vi "rsscope_core_global.vi"() -> ()   [LabVIEW 2014] (continued)
"Descriptive Name"="Search ARINC429 Label Data SSM", "Data Type"=0, "Command"="SEAR:TRIG:ARIN:SSM", "Access"=1, "Range Table"="", "Read Callback"="", "Write Callback"="rsscope_FormatSearchNameInt32_WriteCallback.vi", "Supported Models"="RTO|RTP", "Instrument Options"="", "Flags"=0, "Help"="Sets the sign/status matrix (SSM) bits.\n\nAvailable Repeated Capabilities:\nNone\n\nRemote-control command(s):\nSEARch:TRIGger:ARINc:SSM"}, {"Level"=5, "Class Only"=FALSE, "Identifier"="RSSCOPE_ATTR_SEARCH_ARINC429_LABEL_PATTERN_CONDITION", "Descriptive Name"="Search ARINC429 Label Pattern Condition", "Data Type"=0, "Command"="SEAR:TRIG:ARIN:LAB:COND", "Access"=2, "Range Table"="rsscope_rngProtocolARINC429LabelOperator", "Read Callback"="rsscope_FormatSearchNameInt32_ReadCallback.vi", "Write Callback"="rsscope_FormatSearchNameInt32_WriteCallback.vi", "Supported Models"="RTO|RTP", "Instrument Options"="", "Flags"=0, "Help"="Sets the condition for the label. You can define an exact label or a label range.\n\nAvailable Repeated Capabilities:\nNone\n\nRemote-control command(s):\nSEARch:TRIGger:ARINc:LABel:CONDition"}, {"Level"=5, "Class Only"=FALSE, "Identifier"="RSSCOPE_ATTR_SEARCH_ARINC429_LABEL_PATTERN_MIN", "Descriptive Name"="Search ARINC429 Label Pattern Min", "Data Type"=2, "Command"="SEAR:TRIG:ARIN:LAB:MIN", "Access"=1, "Range Table"="", "Read Callback"="", "Write Callback"="rsscope_FormatSearchNameString_WriteCallback.vi", "Supported Models"="RTO|RTP", "Instrument Options"="", "Flags"=0, "Help"="Defines the minimum bit pattern for the label.\n\nAvailable Repeated Capabilities:\nNone\n\nRemote-control command(s):\nSEARch:TRIGger:ARINc:LABel:MIN"}, {"Level"=5, "Class Only"=FALSE, "Identifier"="RSSCOPE_ATTR_SEARCH_ARINC429_LABEL_PATTERN_MAX", "Descriptive Name"="Search ARINC429 Label Pattern Max", "Data Type"=2, "Command"="SEAR:TRIG:ARIN:LAB:MAX", "Access"=1, "Range Table"="", "Read Callback"="", "Write Callback"="rsscope_FormatSearchNameString_WriteCallback.vi", "Supported Models"="RTO|RTP", "Instrument Options"="", "Flags"=0, "Help"="Sets the end value of a label pattern if &apos;Label Pattern Condition&apos; is set to InRange or OutOfRange.\n\nAvailable Repeated Capabilities:\nNone\n\nRemote-control command(s):\nSEARch:TRIGger:ARINc:LABel:MAX"}, {"Level"=5, "Class Only"=FALSE, "Identifier"="RSSCOPE_ATTR_SEARCH_ARINC429_DATA_PATTERN_CONDITION", "Descriptive Name"="Search ARINC429 Data Pattern Condition", "Data Type"=0, "Command"="SEAR:TRIG:ARIN:DATA:COND", "Access"=2, "Range Table"="rsscope_rngProtocolARINC429DataOperator", "Read Callback"="rsscope_FormatSearchNameInt32_ReadCallback.vi", "Write Callback"="rsscope_FormatSearchNameInt32_WriteCallback.vi", "Supported Models"="RTO|RTP", "Instrument Options"="", "Flags"=0, "Help"="Sets the condition for the data. You can define an exact data patterm or a data range.\n\nAvailable Repeated Capabilities:\nNone\n\nRemote-control command(s):\nSEARch:TRIGger:ARINc:DATA:CONDition"}, {"Level"=5, "Class Only"=FALSE, "Identifier"="RSSCOPE_ATTR_SEARCH_ARINC429_DATA_PATTERN_MIN", "Descriptive Name"="Search ARINC429 Data Pattern Min", "Data Type"=2, "Command"="SEAR:TRIG:ARIN:DATA:MIN", "Access"=1, "Range Table"="", "Read Callback"="", "Write Callback"="rsscope_FormatSearchNameString_WriteCallback.vi", "Supported Models"="RTO|RTP", "Instrument Options"="", "Flags"=0, "Help"="Defines the minimum bit pattern for the data.\n\nAvailable Repeated Capabilities:\nNone\n\nRemote-control command(s):\nSEARch:TRIGger:ARINc:DATA:MIN"}, {"Level"=5, "Class Only"=FALSE, "Identifier"="RSSCOPE_ATTR_SEARCH_ARINC429_DATA_PATTERN_MAX", "Descriptive Name"="Search ARINC429 Data Pattern Max", "Data Type"=2, "Command"="SEAR:TRIG:ARIN:DATA:MAX", "Access"=1, "Range Table"="", "Read Callback"="", "Write Callback"="rsscope_FormatSearchNameString_WriteCallback.vi", "Supported Models"="RTO|RTP", "Instrument Options"="", "Flags"=0, "Help"="Sets the end value of a data pattern if &apos;Data Pattern Condition&apos; is set to InRange or OutOfRange.\n\nAvailable Repeated Capabilities:\nNone\n\nRemote-control command(s):\nSEARch:TRIGger:ARINc:DATA:MAX"}, {"Level"=4, "Class Only"=TRUE, "Identifier"="", "Descriptive Name"="Error Condition", "Data Type"=0, "Command"="", "Access"=0, "Range Table"="", "Read Callback"="", "Write Callback"="", "Supported Models"="", "Instrument Options"="", "Flags"=0, "Help"="Specifies the error conditions to be searched for."}, {"Level"=5, "Class Only"=FALSE, "Identifier"="RSSCOPE_ATTR_SEARCH_ARINC429_ERROR_CODING_ERROR", "Descriptive Name"="Search ARINC429 Error Coding Error", "Data Type"=3, "Command"="SEAR:TRIG:ARIN:ERR:COD", "Access"=2, "Range Table"="", "Read Callback"="rsscope_FormatSearchNameBoolean_ReadCallback.vi", "Write Callback"="rsscope_FormatSearchNameBoolean_WriteCallback.vi", "Supported Models"="RTO|RTP", "Instrument Options"="", "Flags"=0, "Help"="Enables search when a coding error occurs.\n\nAvailable Repeated Capabilities:\nNone\n\nRemote-control command(s):\nSEARch:TRIGger:ARINc:ERRor:CODing"}, {"Level"=5, "Class Only"=FALSE, "Identifier"="RSSCOPE_ATTR_SEARCH_ARINC429_ERROR_PARITY_ERROR", "Descriptive Name"="Search ARINC429 Error Parity Error", "Data Type"=3, "Command"="SEAR:TRIG:ARIN:ERR:PAR", "Access"=2, "Range Table"="", "Read Callback"="rsscope_FormatSearchNameBoolean_ReadCallback.vi", "Write Callback"="rsscope_FormatSearchNameBoolean_WriteCallback.vi", "Supported Models"="RTO|RTP", "Instrument Options"="", "Flags"=0, "Help"="Enables search when a parity error occurs.\n\nAvailable Repeated Capabilities:\nNone\n\nRemote-control command(s):\nSEARch:TRIGger:ARINc:ERRor:PARity"}, {"Level"=5, "Class Only"=FALSE, "Identifier"="RSSCOPE_ATTR_SEARCH_ARINC429_ERROR_TIMING_ERROR", "Descriptive Name"="Search ARINC429 Error Timing Error", "Data Type"=3, "Command"="SEAR:TRIG:ARIN:ERR:TIM", "Access"=2, "Range Table"="", "Read Callback"="rsscope_FormatSearchNameBoolean_ReadCallback.vi", "Write Callback"="rsscope_FormatSearchNameBoolean_WriteCallback.vi", "Supported Models"="RTO|RTP", "Instrument Options"="", "Flags"=0, "Help"="Enables the search for timing errors, when the minimum gap is out of range.\n\nAvailable Repeated Capabilities:\nNone\n\nRemote-control command(s):\nSEARch:TRIGger:ARINc:ERRor:TIMing"}, {"Level"=4, "Class Only"=TRUE, "Identifier"="", "Descriptive Name"="Results", "Data Type"=0, "Command"="", "Access"=0, "Range Table"="", "Read Callback"="", "Write Callback"="", "Supported Models"="", "Instrument Options"="", "Flags"=0, "Help"="Returns the search of the specified word."}, {"Level"=5, "Class Only"=FALSE, "Identifier"="RSSCOPE_ATTR_SEARCH_ARINC429_WORDS_COUNT", "Descriptive Name"="Search ARINC429 Words Count", "Data Type"=0, "Command"="SEAR:RES:ARIN:WCO?", "Access"=0, "Range Table"="", "Read Callback"="rsscope_FormatSearchNameInt32_ReadCallback.vi", "Write Callback"="", "Supported Models"="RTO|RTP", "Instrument Options"="", "Flags"=0, "Help"="Returns the number of decoded words.\n\nAvailable Repeated Capabilities:\nNone\n\nRemote-control command(s):\nSEARch:RESult:ARINc:WCOunt?"}, {"Level"=3, "Class Only"=TRUE, "Identifier"="", "Descriptive Name"="RFFE", "Data Type"=0, "Command"="", "Access"=0, "Range Table"="", "Read Callback"="", "Write Callback"="", "Supported Models"="", "Instrument Options"="", "Flags"=0, "Help"="Configures RFFE search settings."}, {"Level"=4, "Class Only"=FALSE, "Identifier"="RSSCOPE_ATTR_SEARCH_RFFE_TYPE", "Descriptive Name"="Search RFFE Type", "Data Type"=0, "Command"="SEAR:TRIG:RFFE:TYPE", "Access"=2, "Range Table"="rsscope_rngProtocolRFFETriggerType", "Read Callback"="rsscope_FormatSearchNameInt32_ReadCallback.vi", "Write Callback"="rsscope_FormatSearchNameInt32_WriteCallback.vi", "Supported Models"="", "Instrument Options"="K40", "Flags"=0, "Help"="Sets the event to be searched for.\n\nAvailable Repeated Capabilities:\nNone\n\nRemote-control command(s):\nSEARch:TRIGger:RFFE:TYPE"}, {"Level"=4, "Class Only"=FALSE, "Identifier"="RSSCOPE_ATTR_SEARCH_RFFE_INTERRUPT_PATTERN", "Descriptive Name"="Search RFFE Interrupt Pattern", "Data Type"=2, "Command"="SEAR:TRIG:RFFE:INT", "Access"=2, "Range Table"="", "Read Callback"="rsscope_FormatSearchNameString_ReadCallback.vi", "Write Callback"="rsscope_FormatSearchNameString_WriteCallback.vi", "Supported Models"="", "Instrument Options"="K40", "Flags"=0, "Help"="Defines the pattern of the interrrupt identification sequence, which consists of interrupt slots 15 to 0.\n\nAvailable Repeated Capabilities:\nNone\n\nRemote-control command(s):\nSEARch:TRIGger:RFFE:INTerrupt"}, {"Level"=4, "Class Only"=TRUE, "Identifier"="", "Descriptive Name"="Slave Address", "Data Type"=0, "Command"="", "Access"=0, "Range Table"="", "Read Callback"="", "Write Callback"="", "Supported Models"="", "Instrument Options"="", "Flags"=0, "Help"="Searches for a slave address or a slave address range."}, {"Level"=5, "Class Only"=FALSE, "Identifier"="RSSCOPE_ATTR_SEARCH_RFFE_SLAVE_CONDITION", "Descriptive Name"="Search RFFE Slave Condition", "Data Type"=0, "Command"="SEAR:TRIG:RFFE:SADD:COND", "Access"=2, "Range Table"="rsscope_rngProtocolTriggerCondition", "Read Callback"="rsscope_FormatSearchNameInt32_ReadCallback.vi", "Write Callback"="rsscope_FormatSearchNameInt32_WriteCallback.vi", "Supported Models"="", "Instrument Options"="K40", "Flags"=0, "Help"="Sets the operator to search for a specific pattern or a range\n\nAvailable Repeated Capabilities:\nNone\n\nRemote-control command(s):\nSEARch:TRIGger:RFFE:SADD:CONDition"}, {"Level"=5, "Class Only"=FALSE, "Identifier"="RSSCOPE_ATTR_SEARCH_RFFE_SLAVE_MIN", "Descriptive Name"="Search RFFE Slave Min", "Data Type"=2, "Command"="SEAR:TRIG:RFFE:SADD:MIN", "Access"=1, "Range Table"="", "Read Callback"="", "Write Callback"="rsscope_FormatSearchNameString_WriteCallback.vi", "Supported Models"="", "Instrument Options"="K40", "Flags"=0, "Help"="Specifies a pattern, or sets the start value of a pattern range.\n\nAvailable Repeated Capabilities:\nNone\n\nRemote-control command(s):\nSEARch:TRIGger:RFFE:SADD:MIN"}, {"Level"=5, "Class Only"=FALSE, "Identifier"="RSSCOPE_ATTR_SEARCH_RFFE_SLAVE_MAX", "Descriptive Name"="Search RFFE Slave Max", "Data Type"=2, "Command"="SEAR:TRIG:RFFE:SADD:MAX", "Access"=1, "Range Table"="", "Read Callback"="", "Write Callback"="rsscope_FormatSearchNameString_WriteCallback.vi", "Supported Models"="", "Instrument Options"="K40", "Flags"=0, "Help"="Sets the end value of an range if the corresponding condition is set to In Range or Out Of Range.\n\nAvailable Repeated Capabilities:\nNone\n\nRemote-control command(s):\nSEARch:TRIGger:RFFE:SADD:MAX"}, {"Level"=4, "Class Only"=TRUE, "Identifier"="", "Descriptive Name"="Address", "Data Type"=0, "Command"="", "Access"=0, "Range Table"="", "Read Callback"="", "Write Callback"="", "Supported Models"="", "Instrument Options"="", "Flags"=0, "Help"="Searches for a register address or an address range."}, {"Level"=5, "Class Only"=FALSE, "Identifier"="RSSCOPE_ATTR_SEARCH_RFFE_ADDRESS_CONDITION", "Descriptive Name"="Search RFFE Address Condition", "Data Type"=0, "Command"="SEAR:TRIG:RFFE:ADDR:COND", "Access"=2, "Range Table"="rsscope_rngProtocolTriggerCondition", "Read Callback"="rsscope_FormatSearchNameInt32_ReadCallback.vi", "Write Callback"="rsscope_FormatSearchNameInt32_WriteCallback.vi", "Supported Models"="", "Instrument Options"="K40", "Flags"=0, "Help"="Sets the operator to search for a specific pattern or a range\n\nAvailable Repeated Capabilities:\nNone\n\nRemote-control command(s):\nSEARch:TRIGger:RFFE:ADDRess:CONDition"}, {"Level"=5, "Class Only"=FALSE, "Identifier"="RSSCOPE_ATTR_SEARCH_RFFE_ADDRESS_MIN", "Descriptive Name"="Search RFFE Address Min", "Data Type"=2, "Command"="SEAR:TRIG:RFFE:ADDR:MIN", "Access"=1, "Range Table"="", "Read Callback"="", "Write Callback"="rsscope_FormatSearchNameString_WriteCallback.vi", "Supported Models"="", "Instrument Options"="K40", "Flags"=0, "Help"="Specifies a pattern, or sets the start value of a pattern range.\n\nAvailable Repeated Capabilities:\nNone\n\nRemote-control command(s):\nSEARch:TRIGger:RFFE:ADDRess:MIN"}, {"Level"=5, "Class Only"=FALSE, "Identifier"="RSSCOPE_ATTR_SEARCH_RFFE_ADDRESS_MAX", "Descriptive Name"="Search RFFE Address Max", "Data Type"=2, "Command"="SEAR:TRIG:RFFE:ADDR:MAX", "Access"=1, "Range Table"="", "Read Callback"="", "Write Callback"="rsscope_FormatSearchNameString_WriteCallback.vi", "Supported Models"="", "Instrument Options"="K40", "Flags"=0, "Help"="Sets the end value of an range if the corresponding condition is set to In Range or Out Of Range.\n\nAvailable Repeated Capabilities:\nNone\n\nRemote-control command(s):\nSEARch:TRIGger:RFFE:ADDRess:MAX"}, {"Level"=4, "Class Only"=TRUE, "Identifier"="", "Descriptive Name"="Byte Count", "Data Type"=0, "Command"="", "Access"=0, "Range Table"="", "Read Callback"="", "Write Callback"="", "Supported Models"="", "Instrument Options"="", "Flags"=0, "Help"="Searches for a byte count or a byte count range."}, {"Level"=5, "Class Only"=FALSE, "Identifier"="RSSCOPE_ATTR_SEARCH_RFFE_BYTE_COUNT_CONDITION", "Descriptive Name"="Search RFFE Byte Count Condition", "Data Type"=0, "Command"="SEAR:TRIG:RFFE:BCO:COND", "Access"=2, "Range Table"="rsscope_rngProtocolTriggerCondition", "Read Callback"="rsscope_FormatSearchNameInt32_ReadCallback.vi", "Write Callback"="rsscope_FormatSearchNameInt32_WriteCallback.vi", "Supported Models"="", "Instrument Options"="K40", "Flags"=0, "Help"="Sets the operator to search for a specific pattern or a range\n\nAvailable Repeated Capabilities:\nNone\n\nRemote-control command(s):\nSEARch:TRIGger:RFFE:BCOunt:CONDition"}, {"Level"=5, "Class Only"=FALSE, "Identifier"="RSSCOPE_ATTR_SEARCH_RFFE_BYTE_COUNT_MIN", "Descriptive Name"="Search RFFE Byte Count Min", "Data Type"=2, "Command"="SEAR:TRIG:RFFE:BCO:MIN", "Access"=1, "Range Table"="", "Read Callback"="", "Write Callback"="rsscope_FormatSearchNameString_WriteCallback.vi", "Supported Models"="", "Instrument Options"="K40", "Flags"=0, "Help"="Specifies a pattern, or sets the start value of a pattern range.\n\nAvailable Repeated Capabilities:\nNone\n\nRemote-control command(s):\nSEARch:TRIGger:RFFE:BCOunt:MIN"}, {"Level"=5, "Class Only"=FALSE, "Identifier"="RSSCOPE_ATTR_SEARCH_RFFE_BYTE_COUNT_MAX", "Descriptive Name"="Search RFFE Byte Count Max", "Data Type"=2, "Command"="SEAR:TRIG:RFFE:BCO:MAX", "Access"=1, "Range Table"="", "Read Callback"="", "Write Callback"="rsscope_FormatSearchNameString_WriteCallback.vi", "Supported Models"="", "Instrument Options"="K40", "Flags"=0, "Help"="Sets the end value of an range if the corresponding condition is set to In Range or Out Of Range.\n\nAvailable Repeated Capabilities:\nNone\n\nRemote-control command(s):\nSEARch:TRIGger:RFFE:BCOunt:MAX"}, {"Level"=4, "Class Only"=TRUE, "Identifier"="", "Descriptive Name"="Data", "Data Type"=0, "Command"="", "Access"=0, "Range Table"="", "Read Callback"="", "Write Callback"="", "Supported Models"="", "Instrument Options"="", "Flags"=0, "Help"="Searches for a data pattern or an data word range."}, {"Level"=5, "Class Only"=FALSE, "Identifier"="RSSCOPE_ATTR_SEARCH_RFFE_DATA_CONDITION", "Descriptive Name"="Search RFFE Data Condition", "Data Type"=0, "Command"="SEAR:TRIG:RFFE:DATA:DCON", "Access"=2, "Range Table"="rsscope_rngProtocolTriggerCondition", "Read Callback"="rsscope_FormatSearchNameInt32_ReadCallback.vi", "Write Callback"="rsscope_FormatSearchNameInt32_WriteCallback.vi", "Supported Models"="", "Instrument Options"="K40", "Flags"=0, "Help"="Sets the operator to search for a specific pattern or a range\n\nAvailable Repeated Capabilities:\nNone\n\nRemote-control command(s):\nSEARch:TRIGger:RFFE:DATA:DCON"}, {"Level"=5, "Class Only"=FALSE, "Identifier"="RSSCOPE_ATTR_SEARCH_RFFE_DATA_MIN", "Descriptive Name"="Search RFFE Data Min", "Data Type"=2, "Command"="SEAR:TRIG:RFFE:DATA:DMIN", "Access"=1, "Range Table"="", "Read Callback"="", "Write Callback"="rsscope_FormatSearchNameString_WriteCallback.vi", "Supported Models"="", "Instrument Options"="K40", "Flags"=0, "Help"="Specifies a pattern, or sets the start value of a pattern range.\n\nAvailable Repeated Capabilities:\nNone\n\nRemote-control command(s):\nSEARch:TRIGger:RFFE:DATA:DMIN"}, {"Level"=5, "Class Only"=FALSE, "Identifier"="RSSCOPE_ATTR_SEARCH_RFFE_DATA_MAX", "Descriptive Name"="Search RFFE Data Max", "Data Type"=2, "Command"="SEAR:TRIG:RFFE:DATA:DMAX", "Access"=1, "Range Table"="", "Read Callback"="", "Write Callback"="rsscope_FormatSearchNameString_WriteCallback.vi", "Supported Models"="", "Instrument Options"="K40", "Flags"=0, "Help"="Sets the end value of an range if the corresponding condition is set to In Range or Out Of Range.\n\nAvailable Repeated Capabilities:\nNone\n\nRemote-control command(s):\nSEARch:TRIGger:RFFE:DATA:DMAX"}, {"Level"=4, "Class Only"=TRUE, "Identifier"="", "Descriptive Name"="Index", "Data Type"=0, "Command"="", "Access"=0, "Range Table"="", "Read Callback"="", "Write Callback"="", "Supported Models"="", "Instrument Options"="", "Flags"=0, "Help"="Defines which data frames are relevant for the search. The setting is available for all &apos;Extended Register&apos; command sequences, which can transfer more than one data frame. To search for any data byte that fulfills the data pattern settings, set the index to XX."}, {"Level"=5, "Class Only"=FALSE, "Identifier"="RSSCOPE_ATTR_SEARCH_RFFE_INDEX_CONDITION", "Descriptive Name"="Search RFFE Index Condition", "Data Type"=0, "Command"="SEAR:TRIG:RFFE:DATA:ICON", "Access"=2, "Range Table"="rsscope_rngProtocolIndexCondition", "Read Callback"="rsscope_FormatSearchNameInt32_ReadCallback.vi", "Write Callback"="rsscope_FormatSearchNameInt32_WriteCallback.vi", "Supported Models"="", "Instrument Options"="K40", "Flags"=0, "Help"="Sets the operator to search for a specific pattern or a range\n\nAvailable Repeated Capabilities:\nNone\n\nRemote-control command(s):\nSEARch:TRIGger:RFFE:DATA:ICON"}, {"Level"=5, "Class Only"=FALSE, "Identifier"="RSSCOPE_ATTR_SEARCH_RFFE_INDEX_MIN", "Descriptive Name"="Search RFFE Index Min", "Data Type"=0, "Command"="SEAR:TRIG:RFFE:DATA:IMIN", "Access"=2, "Range Table"="", "Read Callback"="rsscope_FormatSearchNameInt32_ReadCallback.vi", "Write Callback"="rsscope_FormatSearchNameInt32_WriteCallback.vi", "Supported Models"="", "Instrument Options"="K40", "Flags"=0, "Help"="Specifies a pattern, or sets the start value of a pattern range.\n\nAvailable Repeated Capabilities:\nNone\n\nRemote-control command(s):\nSEARch:TRIGger:RFFE:DATA:IMIN"}, {"Level"=5, "Class Only"=FALSE, "Identifier"="RSSCOPE_ATTR_SEARCH_RFFE_INDEX_MAX", "Descriptive Name"="Search RFFE Index Max", "Data Type"=0, "Command"="SEAR:TRIG:RFFE:DATA:IMAX", "Access"=2, "Range Table"="", "Read Callback"="rsscope_FormatSearchNameInt32_ReadCallback.vi", "Write Callback"="rsscope_FormatSearchNameInt32_WriteCallback.vi", "Supported Models"="", "Instrument Options"="K40", "Flags"=0, "Help"="Sets the end value of an range if the corresponding condition is set to In Range or Out Of Range.\n\nAvailable Repeated Capabilities:\nNone\n\nRemote-control command(s):\nSEARch:TRIGger:RFFE:DATA:IMAX"}, {"Level"=4, "Class Only"=TRUE, "Identifier"="", "Descriptive Name"="Error Conditions", "Data Type"=0, "Command"="", "Access"=0, "Range Table"="", "Read Callback"="", "Write Callback"="", "Supported Models"="", "Instrument Options"="", "Flags"=0, "Help"="This class configures conditions for Error search."}, {"Level"=5, "Class Only"=FALSE, "Identifier"="RSSCOPE_ATTR_SEARCH_RFFE_ERROR_SCC", "Descriptive Name"="Search RFFE Error SCC", "Data Type"=3, "Command"="SEAR:TRIG:RFFE:ERR:SSC", "Access"=2, "Range Table"="", "Read Callback"="rsscope_FormatSearchNameBoolean_ReadCallback.vi", "Write Callback"="rsscope_FormatSearchNameBoolean_WriteCallback.vi", "Supported Models"="", "Instrument Options"="", "Flags"=0, "Help"="Enables the trigger on an SSC error - when no valid SSC sequence has been found after the idle time.\n\nAvailable Repeated Capabilities:\nNone\n\nRemote-control command(s):\nSEARch:TRIGger:RFFE:ERRor:SSC"}, {"Level"=5, "Class Only"=FALSE, "Identifier"="RSSCOPE_ATTR_SEARCH_RFFE_ERROR_LENGTH", "Descriptive Name"="Search RFFE Error Length", "Data Type"=3, "Command"="SEAR:TRIG:RFFE:ERR:LENG", "Access"=2, "Range Table"="", "Read Callback"="rsscope_FormatSearchNameBoolean_ReadCallback.vi", "Write Callback"="rsscope_FormatSearchNameBoolean_WriteCallback.vi", "Supported Models"="", "Instrument Options"="", "Flags"=0, "Help"="Enables the trigger on a length error - when an incorrect length of the command sequence has been found.\n\nAvailable Repeated Capabilities:\nNone\n\nRemote-control command(s):\nSEARch:TRIGger:RFFE:ERRor:LENGth"}, {"Level"=5, "Class Only"=FALSE, "Identifier"="RSSCOPE_ATTR_SEARCH_RFFE_ERROR_PARITY", "Descriptive Name"="Search RFFE Error Parity", "Data Type"=3, "Command"="SEAR:TRIG:RFFE:ERR:PAR", "Access"=2, "Range Table"="", "Read Callback"="rsscope_FormatSearchNameBoolean_ReadCallback.vi", "Write Callback"="rsscope_FormatSearchNameBoolean_WriteCallback.vi", "Supported Models"="", "Instrument Options"="", "Flags"=0, "Help"="Enables the trigger on incorrect parity bits.\n\nAvailable Repeated Capabilities:\nNone\n\nRemote-control command(s):\nSEARch:TRIGger:RFFE:ERRor:PARity"}, {"Level"=5, "Class Only"=FALSE, "Identifier"="RSSCOPE_ATTR_SEARCH_RFFE_ERROR_GAP_TIME", "Descriptive Name"="Search RFFE Error Gap Time", "Data Type"=3, "Command"="SEAR:TRIG:RFFE:ERR:GAP", "Access"=2, "Range Table"="", "Read Callback"="rsscope_FormatSearchNameBoolean_ReadCallback.vi", "Write Callback"="rsscope_FormatSearchNameBoolean_WriteCallback.vi", "Supported Models"="", "Instrument Options"="", "Flags"=0, "Help"="Enables the search for RFFE gap time error.\n\nAvailable Repeated Capabilities:\nNone\n\nRemote-control command(s):\nSEARch:TRIGger:RFFE:ERRor:GAP"}, {"Level"=5, "Class Only"=FALSE, "Identifier"="RSSCOPE_ATTR_SEARCH_RFFE_ERROR_VERSION", "Descriptive Name"="Search RFFE Error Version", "Data Type"=3, "Command"="SEAR:TRIG:RFFE:ERR:VERS", "Access"=2, "Range Table"="", "Read Callback"="rsscope_FormatSearchNameBoolean_ReadCallback.vi", "Write Callback"="rsscope_FormatSearchNameBoolean_WriteCallback.vi", "Supported Models"="", "Instrument Options"="", "Flags"=0, "Help"="Enables the search for RFFE vresion error.\n\nAvailable Repeated Capabilities:\nNone\n\nRemote-control command(s):\nSEARch:TRIGger:RFFE:ERRor:VERSion"}, {"Level"=4, "Class Only"=TRUE, "Identifier"="", "Descriptive Name"="Results", "Data Type"=0, "Command"="", "Access"=0, "Range Table"="", "Read Callback"="", "Write Callback"="", "Supported Models"="", "Instrument Options"="", "Flags"=0, "Help"="Returns the search result of the specified sequence."}, {"Level"=5, "Class Only"=FALSE, "Identifier"="RSSCOPE_ATTR_SEARCH_RFFE_SEQUENCE_COUNT", "Descriptive Name"="Search RFFE Sequence Count", "Data Type"=0, "Command"="SEAR:RES:RFFE:FCO?", "Access"=0, "Range Table"="", "Read Callback"="rsscope_FormatSearchNameInt32_ReadCallback.vi", "Write Callback"="", "Supported Models"="RTO|RTP", "Instrument Options"="", "Flags"=0, "Help"="Returns the number of command sequences in the current acquisition.\n\nAvailable Repeated Capabilities:\nNone\n\nRemote-control command(s):\nSEARch:RESult:RFFE:FCOunt?"}, {"Level"=3, "Class Only"=TRUE, "Identifier"="", "Descriptive Name"="MDIO", "Data Type"=0, "Command"="", "Access"=0, "Range Table"="", "Read Callback"="", "Write Callback"="", "Supported Models"="", "Instrument Options"="", "Flags"=0, "Help"="Configures MDIO search, option K55."}, {"Level"=4, "Class Only"=FALSE, "Identifier"="RSSCOPE_ATTR_SEARCH_MDIO_TYPE", "Descriptive Name"="Search MDIO Type", "Data Type"=0, "Command"="SEAR:TRIG:MDIO:TYPE", "Access"=2, "Range Table"="rsscope_rngProtocolMDIOTriggerType", "Read Callback"="rsscope_FormatSearchNameInt32_ReadCallback.vi", "Write Callback"="rsscope_FormatSearchNameInt32_WriteCallback.vi", "Supported Models"="", "Instrument Options"="K55", "Flags"=0, "Help"="Selects the search type for MDIO analysis.\n\nAvailable Repeated Capabilities:\nNone\n\nRemote-control command(s):\nSEARch:TRIGger:MDIO:TYPE"}, {"Level"=4, "Class Only"=FALSE, "Identifier"="RSSCOPE_ATTR_SEARCH_MDIO_START_CODE", "Descriptive Name"="Search MDIO Start Code", "Data Type"=0, "Command"="SEAR:TRIG:MDIO:ST", "Access"=2, "Range Table"="rsscope_rngProtocolMDIOTriggerStartCode", "Read Callback"="rsscope_FormatSearchNameInt32_ReadCallback.vi", "Write Callback"="rsscope_FormatSearchNameInt32_WriteCallback.vi", "Supported Models"="", "Instrument Options"="K55", "Flags"=0, "Help"="Selects the start of frame code of the frame pattern.\n\nAvailable Repeated Capabilities:\nNone\n\nRemote-control command(s):\nSEARch:TRIGger:MDIO:ST"}, {"Level"=4, "Class Only"=FALSE, "Identifier"="RSSCOPE_ATTR_SEARCH_MDIO_OPERATION_CODE", "Descriptive Name"="Search MDIO Operation Code", "Data Type"=0, "Command"="SEAR:TRIG:MDIO:FRAM", "Access"=2, "Range Table"="rsscope_rngProtocolMDIOTriggerOperationCode", "Read Callback"="rsscope_FormatSearchNameInt32_ReadCallback.vi", "Write Callback"="rsscope_FormatSearchNameInt32_WriteCallback.vi", "Supported Models"="", "Instrument Options"="K55", "Flags"=0, "Help"="Selects the Type of Frame code (or OP code, OpCode, operation code).\n\nAvailable Repeated Capabilities:\nNone\n\nRemote-control command(s):\nSEARch:TRIGger:MDIO:FRAMetype"}, {"Level"=4, "Class Only"=FALSE, "Identifier"="RSSCOPE_ATTR_SEARCH_MDIO_PHYSICAL_PORT_ADDRESS", "Descriptive Name"="Search MDIO Physical Port Address", "Data Type"=2, "Command"="SEAR:TRIG:MDIO:PHYS", "Access"=1, "Range Table"="", "Read Callback"="", "Write Callback"="rsscope_FormatSearchNameString_WriteCallback.vi", "Supported Models"="", "Instrument Options"="K55", "Flags"=0, "Help"="Sets the physical address (in Clause 22) or port address (in Clause 45) of the frame pattern (5 bits).\n\nAvailable Repeated Capabilities:\nNone\n\nRemote-control command(s):\nSEARch:TRIGger:MDIO:PHYS"}, {"Level"=4, "Class Only"=FALSE, "Identifier"="RSSCOPE_ATTR_SEARCH_MDIO_REGISTER_DEVICE_ADDRESS", "Descriptive Name"="Search MDIO Register Device Address", "Data Type"=2, "Command"="SEAR:TRIG:MDIO:REGI", "Access"=1, "Range Table"="", "Read Callback"="", "Write Callback"="rsscope_FormatSearchNameString_WriteCallback.vi", "Supported Models"="", "Instrument Options"="K55", "Flags"=0, "Help"="Sets the register address (in Clause 22) or device address (in Clause 45) of the frame pattern (5 bits); available only in search type &apos;Data&apos;.\n\nAvailable Repeated Capabilities:\nNone\n\nRemote-control command(s):\nSEARch:TRIGger:MDIO:REGI"}, {"Level"=4, "Class Only"=FALSE, "Identifier"="RSSCOPE_ATTR_SEARCH_MDIO_DATA_ADDRESS_PATTERN", "Descriptive Name"="Search MDIO Data Address Pattern", "Data Type"=2, "Command"="SEAR:TRIG:MDIO:DATA", "Access"=1, "Range Table"="", "Read Callback"="", "Write Callback"="rsscope_FormatSearchNameString_WriteCallback.vi", "Supported Models"="", "Instrument Options"="K55", "Flags"=0, "Help"="Defines the 16-bit payload data pattern (both in Clause 22 or Clause 45) or the address pattern (in Clause 45, only) to search for.\n\nAvailable Repeated Capabilities:\nNone\n\nRemote-control command(s):\nSEARch:TRIGger:MDIO:DATA"}, {"Level"=4, "Class Only"=TRUE, "Identifier"="", "Descriptive Name"="Results", "Data Type"=0, "Command"="", "Access"=0, "Range Table"="", "Read Callback"="", "Write Callback"="", "Supported Models"="", "Instrument Options"="", "Flags"=0, "Help"="Returns the search result of the specified word."}, {"Level"=5, "Class Only"=FALSE, "Identifier"="RSSCOPE_ATTR_SEARCH_MDIO_WORD_COUNT", "Descriptive Name"="Search MDIO Word Count", "Data Type"=0, "Command"="SEAR:RES:MDIO:WCO?", "Access"=0, "Range Table"="", "Read Callback"="rsscope_FormatSearchNameInt32_ReadCallback.vi", "Write Callback"="", "Supported Models"="", "Instrument Options"="K55", "Flags"=0, "Help"="Returns the number of decoded words.\n\nAvailable Repeated Capabilities:\nNone\n\nRemote-control command(s):\nSEARch:RESult:MDIO:WCOunt?"}, {"Level"=3, "Class Only"=TRUE, "Identifier"="", "Descriptive Name"="Ethernet", "Data Type"=0, "Command"="", "Access"=0, "Range Table"="", "Read Callback"="", "Write Callback"="", "Supported Models"="", "Instrument Options"="", "Flags"=0, "Help"="This class contains attributes that configure the  Ethernet protocol variants 10BASE-T and 100BASE-TX.\n\nAttributes in this class require option R&S RTO-K8."}, {"Level"=4, "Class Only"=FALSE, "Identifier"="RSSCOPE_ATTR_SEARCH_ETHERNET_FRAME_ENABLED", "Descriptive Name"="Search Ethernet Frame Enabled", "Data Type"=3, "Command"="SEAR:TRIG:ETH:FRAM:SEL", "Access"=2, "Range Table"="", "Read Callback"="rsscope_FormatSearchNameBoolean_ReadCallback.vi", "Write Callback"="rsscope_FormatSearchNameBoolean_WriteCallback.vi", "Supported Models"="", "Instrument Options"="K8", "Flags"=0, "Help"="Defines, whether a search within a frame shall be activated or not.\n\nAvailable Repeated Capabilities:\nNone\n\nRemote-control command(s):\nSEARch:TRIGger:ETHernet:FRAMe:SELect"}, {"Level"=4, "Class Only"=FALSE, "Identifier"="RSSCOPE_ATTR_SEARCH_ETHERNET_ERROR_ENABLED", "Descriptive Name"="Search Ethernet Error Enabled", "Data Type"=3, "Command"="SEAR:TRIG:ETH:ERR:SEL", "Access"=2, "Range Table"="", "Read Callback"="rsscope_FormatSearchNameBoolean_ReadCallback.vi", "Write Callback"="rsscope_FormatSearchNameBoolean_WriteCallback.vi", "Supported Models"="", "Instrument Options"="K8", "Flags"=0, "Help"="Defines, whether a search for an error condition shall be activated or not.\n\nAvailable Repeated Capabilities:\nNone\n\nRemote-control command(s):\nSEARch:TRIGger:ETHernet:ERRor:SELect"}, {"Level"=4, "Class Only"=TRUE, "Identifier"="", "Descriptive Name"="Destination Address", "Data Type"=0, "Command"="", "Access"=0, "Range Table"="", "Read Callback"="", "Write Callback"="", "Supported Models"="", "Instrument Options"="", "Flags"=0, "Help"="To search for a destination address, an address pattern or optionally an address range have to be specified."}, {"Level"=5, "Class Only"=FALSE, "Identifier"="RSSCOPE_ATTR_SEARCH_ETHERNET_DESTINATION_ADDRESS_CONDITION", "Descriptive Name"="Search Ethernet Destination Address Condition", "Data Type"=0, "Command"="SEAR:TRIG:ETH:FRAM:DCON", "Access"=2, "Range Table"="rsscope_rngProtocolTriggerCondition", "Read Callback"="rsscope_FormatSearchNameInt32_ReadCallback.vi", "Write Callback"="rsscope_FormatSearchNameInt32_WriteCallback.vi", "Supported Models"="", "Instrument Options"="K8", "Flags"=0, "Help"="Defines the operator to search a specific destination address within a frame.\n\nAvailable Repeated Capabilities:\nNone\n\nRemote-control command(s):\nSEARch:TRIGger:ETHernet:FRAMe:DCONdition"}, {"Level"=5, "Class Only"=FALSE, "Identifier"="RSSCOPE_ATTR_SEARCH_ETHERNET_DESTINATION_ADDRESS_MIN", "Descriptive Name"="Search Ethernet Destination Address Min", "Data Type"=2, "Command"="SEAR:TRIG:ETH:FRAM:DMIN", "Access"=1, "Range Table"="", "Read Callback"="", "Write Callback"="rsscope_FormatSearchNameString_WriteCallback.vi", "Supported Models"="", "Instrument Options"="K8", "Flags"=0, "Help"="Defines a destination address, or sets the start value of a destination address range.\n\nAvailable Repeated Capabilities:\nNone\n\nRemote-control command(s):\nSEARch:TRIGger:ETHernet:FRAMe:DMIN"}, {"Level"=5, "Class Only"=FALSE, "Identifier"="RSSCOPE_ATTR_SEARCH_ETHERNET_DESTINATION_ADDRESS_MAX", "Descriptive Name"="Search Ethernet Destination Address Max", "Data Type"=2, "Command"="SEAR:TRIG:ETH:FRAM:DMAX", "Access"=1, "Range Table"="", "Read Callback"="", "Write Callback"="rsscope_FormatSearchNameString_WriteCallback.vi", "Supported Models"="", "Instrument Options"="K8", "Flags"=0, "Help"="Sets the end value of a destination address range if the corresponding condition is set to In Range or Out Of Range.\n\nAvailable Repeated Capabilities:\nNone\n\nRemote-control command(s):\nSEARch:TRIGger:ETHernet:FRAMe:DMAX"}, {"Level"=4, "Class Only"=TRUE, "Identifier"="", "Descriptive Name"="Source Address", "Data Type"=0, "Command"="", "Access"=0, "Range Table"="", "Read Callback"="", "Write Callback"="", "Supported Models"="", "Instrument Options"="", "Flags"=0, "Help"="To search for a source address, an address pattern or optionally an address range have to be specified."}, {"Level"=5, "Class Only"=FALSE, "Identifier"="RSSCOPE_ATTR_SEARCH_ETHERNET_SOURCE_ADDRESS_CONDITION", "Descriptive Name"="Search Ethernet Source Address Condition", "Data Type"=0, "Command"="SEAR:TRIG:ETH:FRAM:SCON", "Access"=2, "Range Table"="rsscope_rngProtocolTriggerCondition", "Read Callback"="rsscope_FormatSearchNameInt32_ReadCallback.vi", "Write Callback"="rsscope_FormatSearchNameInt32_WriteCallback.vi", "Supported Models"="", "Instrument Options"="K8", "Flags"=0, "Help"="Defines the operator to search a specific source address within a frame.\n\nAvailable Repeated Capabilities:\nNone\n\nRemote-control command(s):\nSEARch:TRIGger:ETHernet:FRAMe:SCONdition"}, {"Level"=5, "Class Only"=FALSE, "Identifier"="RSSCOPE_ATTR_SEARCH_ETHERNET_SOURCE_ADDRESS_MIN", "Descriptive Name"="Search Ethernet Source Address Min", "Data Type"=2, "Command"="SEAR:TRIG:ETH:FRAM:SMIN", "Access"=1, "Range Table"="", "Read Callback"="", "Write Callback"="rsscope_FormatSearchNameString_WriteCallback.vi", "Supported Models"="", "Instrument Options"="K8", "Flags"=0, "Help"="Defines a destination address, or sets the start value of a source address range.\n\nAvailable Repeated Capabilities:\nNone\n\nRemote-control command(s):\nSEARch:TRIGger:ETHernet:FRAMe:SMIN"}, {"Level"=5, "Class Only"=FALSE, "Identifier"="RSSCOPE_ATTR_SEARCH_ETHERNET_SOURCE_ADDRESS_MAX", "Descriptive Name"="Search Ethernet Source Address Max", "Data Type"=2, "Command"="SEAR:TRIG:ETH:FRAM:SMAX", "Access"=1, "Range Table"="", "Read Callback"="", "Write Callback"="rsscope_FormatSearchNameString_WriteCallback.vi", "Supported Models"="", "Instrument Options"="K8", "Flags"=0, "Help"="Sets the end value of a source address range if the corresponding condition is set to In Range or Out Of Range.\n\nAvailable Repeated Capabilities:\nNone\n\nRemote-control command(s):\nSEARch:TRIGger:ETHernet:FRAMe:SMAX"}, {"Level"=4, "Class Only"=TRUE, "Identifier"="", "Descriptive Name"="Type Length", "Data Type"=0, "Command"="", "Access"=0, "Range Table"="", "Read Callback"="", "Write Callback"="", "Supported Models"="", "Instrument Options"="", "Flags"=0, "Help"="To search for a frame length or frame type, a type/length pattern or optionally a range of type/length patterns have to be specified."}, {"Level"=5, "Class Only"=FALSE, "Identifier"="RSSCOPE_ATTR_SEARCH_ETHERNET_TYPE_LENGTH_CONDITION", "Descriptive Name"="Search Ethernet Type Length Condition", "Data Type"=0, "Command"="SEAR:TRIG:ETH:FRAM:TCON", "Access"=2, "Range Table"="rsscope_rngProtocolTriggerCondition", "Read Callback"="rsscope_FormatSearchNameInt32_ReadCallback.vi", "Write Callback"="rsscope_FormatSearchNameInt32_WriteCallback.vi", "Supported Models"="", "Instrument Options"="K8", "Flags"=0, "Help"="Defines the operator to search for a specific frame length or type.\n\nAvailable Repeated Capabilities:\nNone\n\nRemote-control command(s):\nSEARch:TRIGger:ETHernet:FRAMe:TCONdition"}, {"Level"=5, "Class Only"=FALSE, "Identifier"="RSSCOPE_ATTR_SEARCH_ETHERNET_TYPE_LENGTH_MIN", "Descriptive Name"="Search Ethernet Type Length Min", "Data Type"=2, "Command"="SEAR:TRIG:ETH:FRAM:TMIN", "Access"=1, "Range Table"="", "Read Callback"="", "Write Callback"="rsscope_FormatSearchNameString_WriteCallback.vi", "Supported Models"="", "Instrument Options"="K8", "Flags"=0, "Help"="Defines a frame length/type, or sets the start value for a range of frame lengths/types.\n\nAvailable Repeated Capabilities:\nNone\n\nRemote-control command(s):\nSEARch:TRIGger:ETHernet:FRAMe:TMIN"}, {"Level"=5, "Class Only"=FALSE, "Identifier"="RSSCOPE_ATTR_SEARCH_ETHERNET_TYPE_LENGTH_MAX", "Descriptive Name"="Search Ethernet Type Length Max", "Data Type"=2, "Command"="SEAR:TRIG:ETH:FRAM:TMAX", "Access"=1, "Range Table"="", "Read Callback"="", "Write Callback"="rsscope_FormatSearchNameString_WriteCallback.vi", "Supported Models"="", "Instrument Options"="K8", "Flags"=0, "Help"="Sets the end value of a range of frame lengths/types if the corresponding condition is set to In Range or Out Of Range.\n\nAvailable Repeated Capabilities:\nNone\n\nRemote-control command(s):\nSEARch:TRIGger:ETHernet:FRAMe:TMAX"}, {"Level"=4, "Class Only"=TRUE, "Identifier"="", "Descriptive Name"="Frame Check", "Data Type"=0, "Command"="", "Access"=0, "Range Table"="", "Read Callback"="", "Write Callback"="", "Supported Models"="", "Instrument Options"="", "Flags"=0, "Help"="To search for a specific pattern, this pattern or optionally a range of patterns have to be specified."}, {"Level"=5, "Class Only"=FALSE, "Identifier"="RSSCOPE_ATTR_SEARCH_ETHERNET_FRAME_CHECK_CONDITION", "Descriptive Name"="Search Ethernet Frame Check Condition", "Data Type"=0, "Command"="SEAR:TRIG:ETH:FRAM:CCON", "Access"=2, "Range Table"="rsscope_rngProtocolTriggerCondition", "Read Callback"="rsscope_FormatSearchNameInt32_ReadCallback.vi", "Write Callback"="rsscope_FormatSearchNameInt32_WriteCallback.vi", "Supported Models"="", "Instrument Options"="K8", "Flags"=0, "Help"="Defines the operator to search for a Cyclic Redundancy Code (CRC, or frame check) error condition within a frame.\n\nAvailable Repeated Capabilities:\nNone\n\nRemote-control command(s):\nSEARch:TRIGger:ETHernet:FRAMe:CCONdition"}, {"Level"=5, "Class Only"=FALSE, "Identifier"="RSSCOPE_ATTR_SEARCH_ETHERNET_FRAME_CHECK_MIN", "Descriptive Name"="Search Ethernet Frame Check Min", "Data Type"=2, "Command"="SEAR:TRIG:ETH:FRAM:CMIN", "Access"=1, "Range Table"="", "Read Callback"="", "Write Callback"="rsscope_FormatSearchNameString_WriteCallback.vi", "Supported Models"="", "Instrument Options"="K8", "Flags"=0, "Help"="Defines a CRC error condition pattern, or sets the start value of such a pattern.\n\nAvailable Repeated Capabilities:\nNone\n\nRemote-control command(s):\nSEARch:TRIGger:ETHernet:FRAMe:CMIN"}, {"Level"=5, "Class Only"=FALSE, "Identifier"="RSSCOPE_ATTR_SEARCH_ETHERNET_FRAME_CHECK_MAX", "Descriptive Name"="Search Ethernet Frame Check Max", "Data Type"=2, "Command"="SEAR:TRIG:ETH:FRAM:CMAX", "Access"=1, "Range Table"="", "Read Callback"="", "Write Callback"="rsscope_FormatSearchNameString_WriteCallback.vi", "Supported Models"="", "Instrument Options"="K8", "Flags"=0, "Help"="Sets the end value of a CRC error condition pattern if the corresponding condition is set to In Range or Out Of Range.\n\nAvailable Repeated Capabilities:\nNone\n\nRemote-control command(s):\nSEARch:TRIGger:ETHernet:FRAMe:CMAX"}, {"Level"=4, "Class Only"=TRUE, "Identifier"="", "Descriptive Name"="Error Conditions", "Data Type"=0, "Command"="", "Access"=0, "Range Table"="", "Read Callback"="", "Write Callback"="", "Supported Models"="", "Instrument Options"="", "Flags"=0, "Help"="This class configures conditions for Error search."}, {"Level"=5, "Class Only"=FALSE, "Identifier"="RSSCOPE_ATTR_SEARCH_ETHERNET_ERROR_PREAMBLE", "Descriptive Name"="Search Ethernet Error Preamble", "Data Type"=3, "Command"="SEAR:TRIG:ETH:ERR:PRE", "Access"=2, "Range Table"="", "Read Callback"="rsscope_FormatSearchNameBoolean_ReadCallback.vi", "Write Callback"="rsscope_FormatSearchNameBoolean_WriteCallback.vi", "Supported Models"="", "Instrument Options"="K8", "Flags"=0, "Help"="Defines, whether a search for any preamble error shall be activated or not.\n\nAvailable Repeated Capabilities:\nNone\n\nRemote-control command(s):\nSEARch:TRIGger:ETHernet:ERRor:PREamble"}, {"Level"=5, "Class Only"=FALSE, "Identifier"="RSSCOPE_ATTR_SEARCH_ETHERNET_ERROR_LENGTH", "Descriptive Name"="Search Ethernet Error Length", "Data Type"=3, "Command"="SEAR:TRIG:ETH:ERR:LENG", "Access"=2, "Range Table"="", "Read Callback"="rsscope_FormatSearchNameBoolean_ReadCallback.vi", "Write Callback"="rsscope_FormatSearchNameBoolean_WriteCallback.vi", "Supported Models"="", "Instrument Options"="K8", 
